vi "UTILITY Find Newfi Device.vi"(8 "error in (no error)":errorcluster, 11 "Board ID Config":string) -> (0 "error out":errorcluster, 1 "Array of Newfi Devices":string[](array[string]), 2 "Number of Newfi's":i32, 3 "Current Board Index":i32)   [LabVIEW 2016]
uses:
  <vilib>/Utility/error.llb/whitespace.ctl
  C:/Technology Lab/NI-2010/Trunk/Utility/LabVIEW GEA2 Toolkit v1.0.0.0/Appliance.NET/GeaCommunication.Usb.dll
  LabVIEW GEA2 Toolkit v1.0.0.0/Appliance.NET/GeaCommunication.Usb.dll
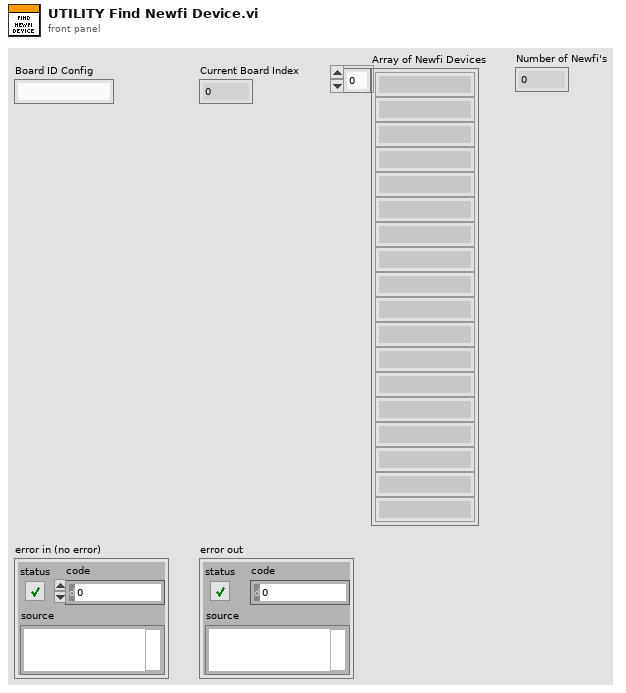
[diagram p1: front panel]
types:
  T1 = typedef "whitespace.ctl" = u16
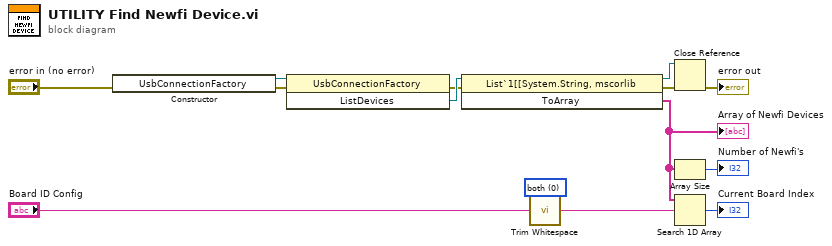
[diagram p0: block diagram]
diagram:
  w13 = T1 0 items=["both", "start of string", "end of string"] ("location (both)")
  n1 = constructor class="UsbConnectionFactory"(error in="error in (no error)") -> (reference out=w3:refnum<k24>, error out=w11:errorcluster)  [unwired: 2 in, 1 out]
  n2 = invoke class="UsbConnectionFactory" method="ListDevices"(reference=w3, error in=w11) -> (error out=w4:errorcluster, "ListDevices"=w5:refnum<k24>)  [unwired: 1 in, 1 out]
  n3 = invoke class="List`1[[System.String, mscorlib" method="ToArray"(reference=w5, error in=w4) -> (reference out=w8:refnum<k24>, error out=w9:errorcluster, "ToArray"=w2:string[])  [unwired: 1 in]
  "Array of Newfi Devices" <- w2
  n4 = call <vilib>:"Trim Whitespace.vi"("string"="Board ID Config", "location (both)"=w13) -> ("trimmed string"=w12:string)
  n5 = Close Reference(reference=w8, error in (no error)=w9) -> (error out=→"error out":errorcluster)
  n6 = Array Size(array=w2) -> (size(s)=→"Number of Newfi's":i32)
  n7 = Search 1D Array(1D array=w2, element=w12) -> (index of element=→"Current Board Index":i32)  [unwired: 1 in]
